vi "roi custom.vi"(7 "Table":string[][](table), 8 "Error In":errorcluster, 9 "Cluster roi in":T1, 10 "List ROI In":dbl[][](array[numeric])=[[0.3012553778449383, 212.0, 307.0, 0.5262321564627634, 0.8298391617333317], [0.2179900662742938, 553.0, 621.0, 1.6160215122234347, 1.8333402107328942], [0.22189128311116604, 733.0, 803.0, 2.191276890630827, 2.414987315567035], [0.23707568654928451, 828.0, 903.0, 2.4948838959013955, 2.7345736369044755], [0.2412265359516473, 934.0, 1009.0, 2.8336453965190818, 3.0733351375221623], [0.2513822152119088, 1043.0, 1122.0, 3.1819944867768917, 3.4344676806334697], [0.26973683252141784, 1160.0, 1245.0, 3.5559104827416967, 3.827558855878521], [0.2678717881623769, 1262.0, 1346.0, 3.881888530505886, 4.150341040429336], [0.3655354172589007, 1993.0, 2108.0, 6.218064539482575, 6.585588809020631], [0.7506683128748562, 2149.0, 2384.0, 6.716619200768982, 7.467647055911966], [2.1181627125190436, 2011.0, 2674.0, 6.275590077323314, 8.394447387790542], [0.43800378659372247, 2675.0, 2812.0, 8.397643251003917, 8.835476511236209], [0.5591543936369769, 3248.0, 3423.0, 10.228872872267448, 10.78814893460797], [2.0749877811247526, 3255.0, 3905.0, 10.25124391476107, 12.328555003454431], [0.6538766230325155, 3874.0, 4079.0, 12.229483243839825, 12.884635202581578], [1.665395130354023, 3928.0, 4449.0, 12.402059857362042, 14.067104591530107], [2.158726430729142, 3864.0, 4539.0, 12.197524611706081, 14.354732280733803], [2.8437575673503135, 3761.0, 4651.0, 11.868350700728518, 14.712668960631735], [1.0965176651033317, 4263.0, 4606.0, 13.472674033842468, 14.568855116029887], [1.057086223423736, 4461.0, 4792.0, 14.1054549500906, 15.163285673717526], [3.6014808329940444, 4123.0, 5250.0, 13.025253183970051, 16.626991025443004], [1.8340552896834679, 4464.0, 5038.0, 14.115042539730723, 15.94946802420763], [0.8581987727342874, 5092.0, 5361.0, 16.122044637729847, 16.981731842127562], [0.7310431391128931, 5331.0, 5560.0, 16.88585594572633, 17.617708621589067], [1.0786009722571657, 5670.0, 6007.0, 17.96925357506025, 19.046259477967425], [1.4137366363648523, 5888.0, 6330.0, 18.665951755575872, 20.078523295887358], [0.9906741851963119, 7611.0, 7921.0, 24.172424072219968, 25.16314166836603]], 11 "Spectrum In":cluster{"Locations":dbl[], "Amplitudes":dbl[]}) -> (0 "Error Out":errorcluster, 2 "Cluster roi out":T1, 3 "List ROI Out":dbl[][](array[numeric]))   [LabVIEW 2023]
uses:
  <vilib>/Utility/miscctls.llb/LVRangeTypeDef.ctl
panel:
  out "subarray":dbl[](array[numeric])
  in  "Stop Button":bool
  out "Spectrum":cluster{"Locations":dbl[], "Amplitudes":dbl[]}[](graph)
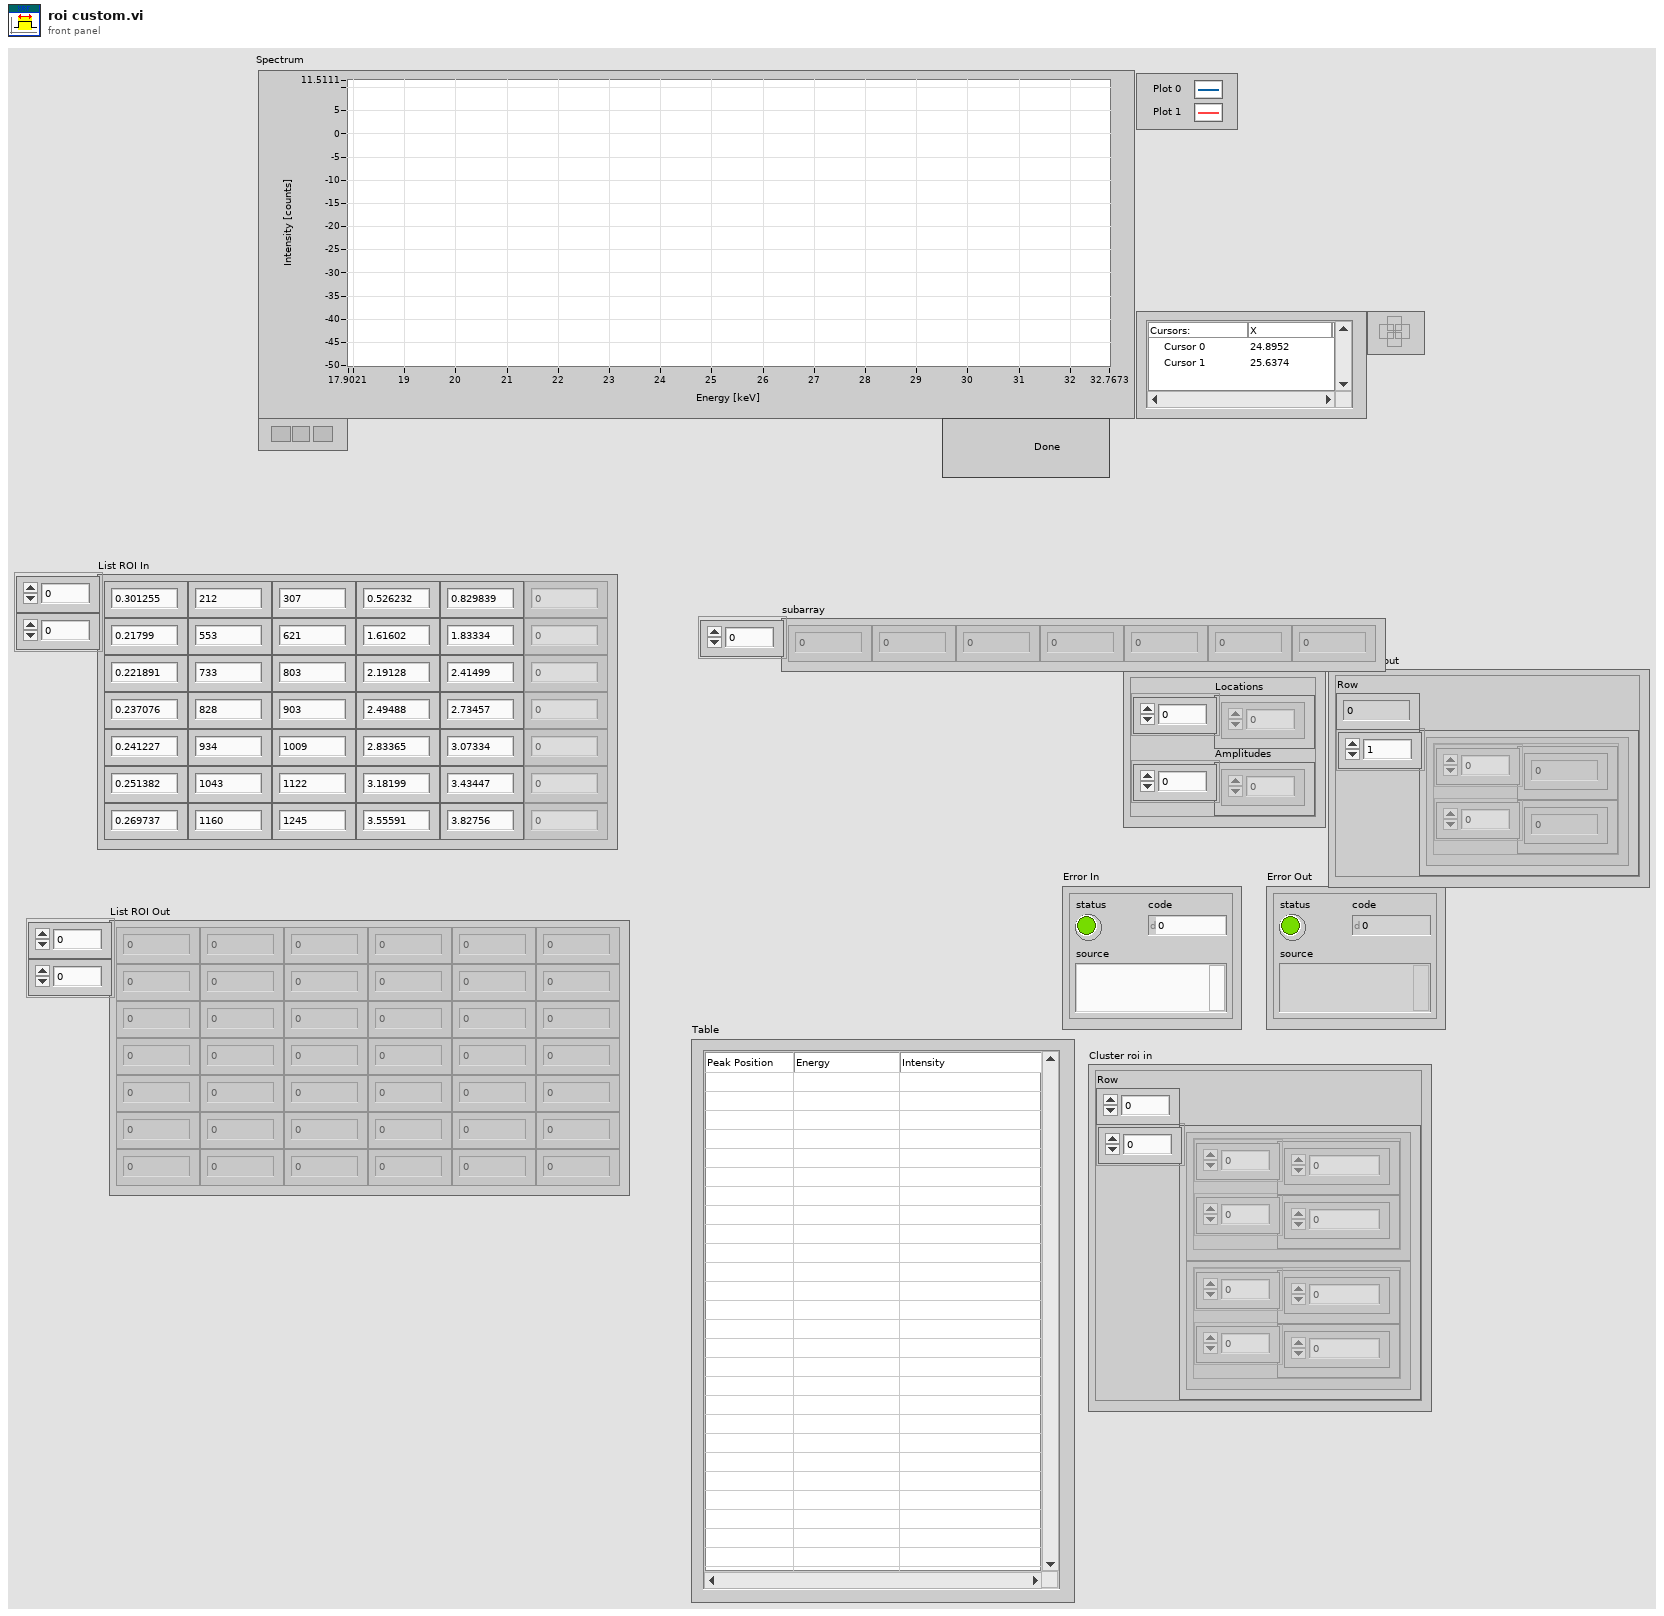
[diagram p1: front panel]
types:
  T1 = cluster{"Row":i32, "Array":cluster{"Array":dbl[], "Array":dbl[]}[]}
  T2 = cluster{"Ch0":dbl, "Ch1":dbl, "E0":dbl, "E1":dbl}
  T3 = typedef "LVRangeTypeDef.ctl" = cluster{"Minimum":dbl, "Maximum":dbl, "Increment":dbl, "Minor Increment":dbl, "Start":dbl}
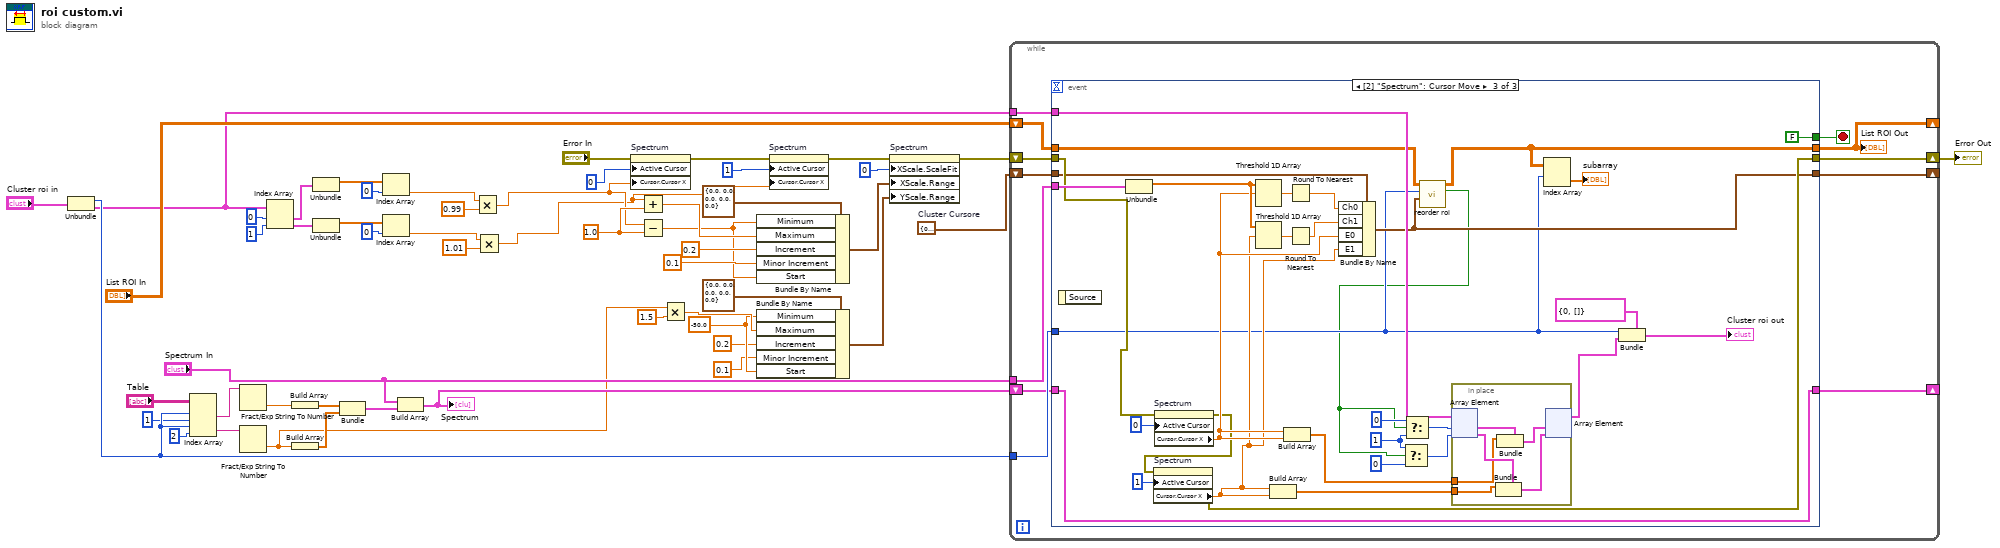
[diagram p0: block diagram]
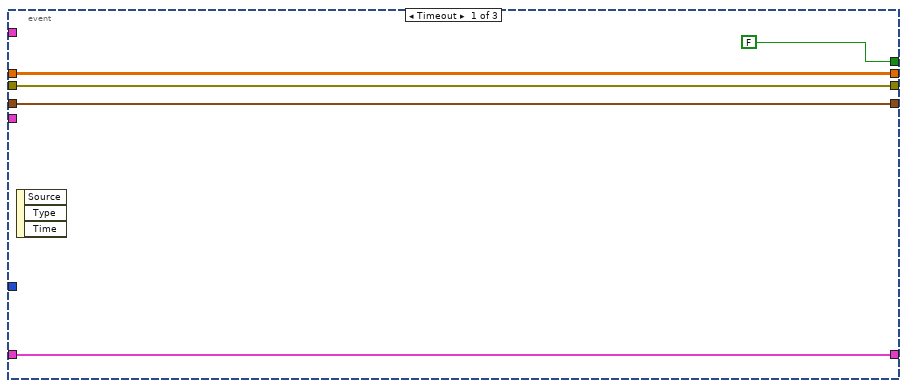
[diagram p2: hidden frame]
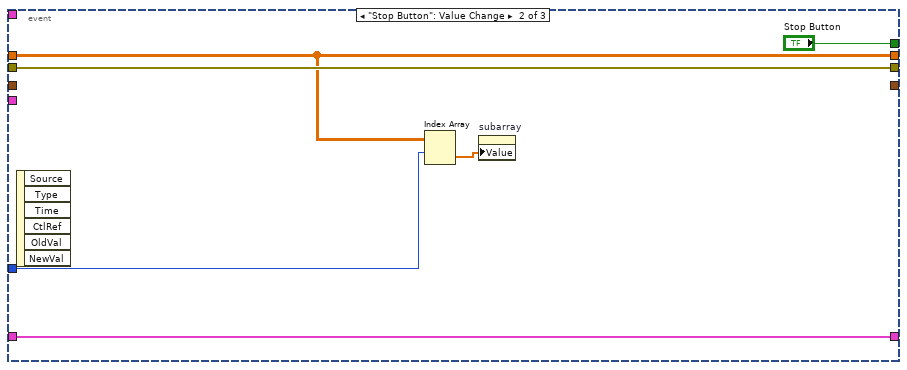
[diagram p3: hidden frame]
diagram:
  w8 = T2 {"Ch0"=0.0, "Ch1"=0.0, "E0"=0.0, "E1"=0.0}  # Cluster Cursore
  w25 = -50.0 ("Minimum")
  w37 = 1.0 ("y")
  n1 = Unbundle("Cluster roi in") -> ("Row"=w20:i32, "Array"=w10:cluster{"Array":dbl[], "Array":dbl[]}[])
  n2 = Index Array(array="Table", index (row) #1=w20, index (col) #1=1, index (row) #2=w20, index (col) #2=2) -> (element #1=w17:string, element #2=w16:string)
  n3 = Fract/Exp String To Number(string=w17) -> (number=w13:dbl)  [unwired: 3 in, 1 out]
  n4 = Fract/Exp String To Number(string=w16) -> (number=w7:dbl)  [unwired: 3 in, 1 out]
  n5 = Index Array(array=w10, index #1=0 ("index"), index #2=1 ("index")) -> (element #1=w50:cluster{"Array":dbl[], "Array":dbl[]}, element #2=w49:cluster{"Array":dbl[], "Array":dbl[]})
  n6 = Build Array(w13) -> (w12:dbl[])
  n7 = Build Array(w7) -> (w11:dbl[])
  n8 = Unbundle(w50) -> ("Array"=w48:dbl[])  [unwired: 1 out]
  n9 = Unbundle(w49) -> ("Array"=w45:dbl[])  [unwired: 1 out]
  n10 = Bundle(w12, w11) -> (w14:cluster{dbl[], dbl[]})  [unwired: 1 in]
  n11 = Index Array(array=w48, index=0) -> (element=w4:dbl)
  n12 = Index Array(array=w45, index=0) -> (element=w2:dbl)
  n13 = Build Array("Spectrum In", w14) -> (w9:cluster{"Locations":dbl[], "Amplitudes":dbl[]}[])
  "Spectrum" <- w9
  n14 = Multiply(x=w4, y=0.99) -> (x*y=w3:dbl)
  n15 = Multiply(x=w2, y=1.01) -> (x*y=w1:dbl)
  n16 = property on="Spectrum" class="XYGraph (strict)"(error in="Error In", "Active Cursor"=u32 0, "Cursor.Cursor X"=w3) -> (error out=w43:errorcluster)  [unwired: 1 in, 1 out]
  n17 = Add(x=w1, y=w37) -> (x+y=w38:dbl)
  n18 = Subtract(x=w3, y=w37) -> (x-y=w26:dbl)
  n19 = Multiply(x=w7, y=1.5) -> (x*y=w35:dbl)
  n20 = Bundle By Name(cluster=T3 {"Minimum"=0.0, "Maximum"=0.0, "Increment"=0.0, "Minor Increment"=0.0, "Start"=0.0} ("output cluster"), "Minimum"=w26, "Maximum"=w38, "Increment"=0.2, "Minor Increment"=0.1 ("Increment"), "Start"=w26) -> (w32:T3)
  n21 = Bundle By Name(cluster=T3 {"Minimum"=0.0, "Maximum"=0.0, "Increment"=0.0, "Minor Increment"=0.0, "Start"=0.0} ("Y Scale.Range"), "Minimum"=w25, "Maximum"=w35, "Increment"=0.2, "Minor Increment"=0.1 ("Increment"), "Start"=w25) -> (w22:T3)
  n22 = property on="Spectrum" class="XYGraph (strict)"(error in=w43, "Active Cursor"=u32 1, "Cursor.Cursor X"=w1) -> (error out=w39:errorcluster)  [unwired: 1 in, 1 out]
  n23 = property on="Spectrum" class="XYGraph (strict)"(error in=w39, "XScale.ScaleFit"=u8 0 ("X Scale.Scale Fit"), "XScale.Range"=w32, "YScale.Range"=w22) -> (error out=w29:errorcluster)  [unwired: 1 in, 1 out]
  n24 = while {
    shift-right: [w62] -> w40
    shift-left: w29 -> [w64]
    shift-right: [w59] -> _
    shift-left: "List ROI In" -> [w63]
    tunnel: "Spectrum In" -> [w61]
    tunnel: w20 -> [w60]
    tunnel: w10 -> [w58]
    shift-right: [w56] -> _
    shift-left: w9 -> [w57]
    shift-right: [w55] -> _
    shift-left: w8 -> [w54]
    stop <- w65 stop-if-true
    n25 = event shown="[2] \"Spectrum\": Cursor Move" {
      selector: _ -> [_ _ _]
      dyn-events: _ -> [_ _ _]
      timeout: _ -> [_ _ _]
      tunnel: [FALSE ("Stop Button") "Stop Button" FALSE ("Stop Button")] -> w65
      tunnel: w64 -> [w69 w75 w103]
      tunnel: [w66 w71 w79] -> w59
      tunnel: w63 -> [w66 w71 w81]
      tunnel: [w69 w75 w102] -> w62
      tunnel: w61 -> [_ _ w108]
      tunnel: w60 -> [_ w72 w78]
      tunnel: w58 -> [_ _ w92]
      tunnel: w57 -> [w68 w74 w101]
      tunnel: [w68 w74 w101] -> w56
      tunnel: [w67 _ w82] -> w55
      tunnel: w54 -> [w67 _ w93]
      event Timeout {
        n26 = event-data() -> ()  [unwired: 1 in, 3 out]
      }
      event "Stop Button": Value Change {
        n27 = event-data() -> ()  [unwired: 1 in, 6 out]
        n28 = Index Array(array=w71, index (row)=w72) -> (element=w73:dbl[])  [unwired: 1 in]
        n29 = property on="subarray" class="Arr (strict)"("Value"=w73) -> ()  [unwired: 2 in, 2 out]
      }
      event "Spectrum": Cursor Move {
        w90 = 1 ("index")
        n30 = event-data() -> ()  [unwired: 1 in, 1 out]
        n31 = Unbundle(w108) -> ("Locations"=w98:dbl[])  [unwired: 1 out]
        n32 = property on="Spectrum" class="XYGraph (strict)"(error in=w103, "Active Cursor"=u32 0) -> (error out=w86:errorcluster, "Cursor.Cursor X"=w95:dbl)  [unwired: 1 in, 1 out]
        n33 = property on="Spectrum" class="XYGraph (strict)"(error in=w86, "Active Cursor"=u32 1) -> (error out=w102:errorcluster, "Cursor.Cursor X"=w94:dbl)  [unwired: 1 in, 1 out]
        n34 = Threshold 1D Array(2:w95, 3:w98) -> (0:w100:dbl)  [unwired: 1 in]
        n35 = Threshold 1D Array(2:w94, 3:w98) -> (0:w99:dbl)  [unwired: 1 in]
        n36 = Build Array(w94, w94) -> (w84:dbl[])
        n37 = Build Array(w95, w95) -> (w85:dbl[])
        n38 = Round To Nearest(number=w100) -> (nearest integer value=w97:dbl)
        n39 = Round To Nearest(number=w99) -> (nearest integer value=w96:dbl)
        n40 = Bundle By Name(cluster=w93, "Ch0"=w97, "Ch1"=w96, "E0"=w95, "E1"=w94) -> (w82:T2)
        n41 = call "reorder roi.vi"("Cluster Cursori"=w82, "Peak"=w78, "List ROI In in"=w81) -> ("invert?"=w77:bool, "List ROI In out"=w79:dbl[][])  [unwired: 7 in]
        n42 = Select(t=w90, s=w77, f=0 ("index")) -> (s? t:f=w87:i32)
        n43 = Select(t=0 ("index"), s=w77, f=w90) -> (s? t:f=w88:i32)
        n44 = in-place {
          in-place-border: w85 -> [w111]
          in-place-border: w84 -> [w110]
          n45 = in-place-array #1(w92, w88, w87) -> (w115:cluster{"Array":dbl[], "Array":dbl[]}, w114:cluster{"Array":dbl[], "Array":dbl[]})
          n46 = Bundle(cluster=w114, "Array"=w110) -> (w112:cluster{"Array":dbl[], "Array":dbl[]})  [unwired: 1 in]
          n47 = Bundle(cluster=w115, "Array"=w111) -> (w113:cluster{"Array":dbl[], "Array":dbl[]})  [unwired: 1 in]
          n48 = in-place-array #1(w113, w112) -> (w83:cluster{"Array":dbl[], "Array":dbl[]}[])  [unwired: 2 out]
        }
        n49 = Index Array(array=w79, index (row)=w78) -> (element=→"subarray":dbl[])  [unwired: 1 in]
        n50 = Bundle(cluster=cluster{i32, cluster{dbl[], dbl[]}[]} {0, []}, w78, w83) -> (→"Cluster roi out":cluster{i32, cluster{dbl[], dbl[]}[]})
      }
    }
    "List ROI Out" <- w59
  }
  "Error Out" <- w40
